vi "Write.vi"(8 "error in (no error)":errorcluster, 10 "write buffer":string, 11 "MODBUS in":refnum<class "PL Modbus Client.lvclass">) -> (0 "error out":errorcluster, 3 "MODBUS out":refnum<class "PL Modbus Client.lvclass">)   [LabVIEW 2015, in "PL Modbus Client.lvclass"]
doc: "Writes bytes to specified interface."
uses:
  PL Modbus Client.lvclass
  PL Modbus Client.lvclass/PL Modbus Client.ctl
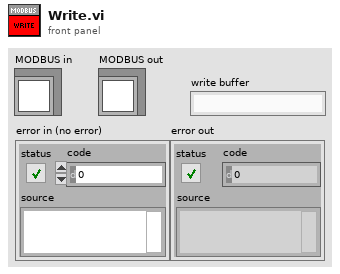
[diagram p1: front panel]
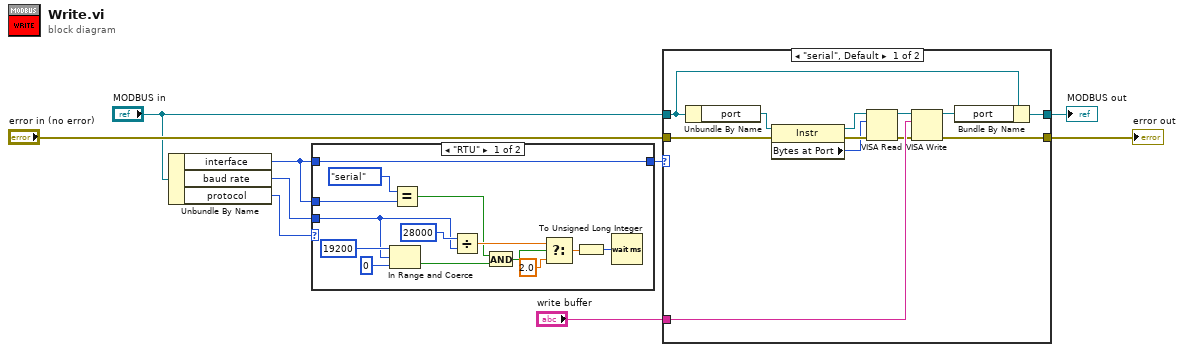
[diagram p0: block diagram]
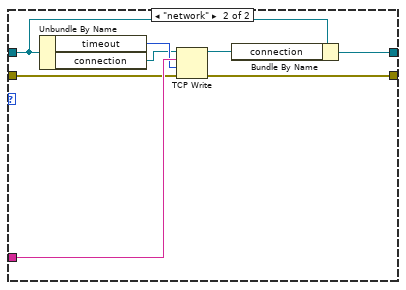
[diagram p3: hidden frame]
diagram:
  n1 = Unbundle By Name("MODBUS in") -> ("interface"=w4:enum16{"serial", "network"}, "baud rate"=w5:u32, "protocol"=w6:enum16{"RTU", "ASCII", "TCP"})
  n2 = case shown="\"RTU\"" w6 {
    tunnel: w5 -> [w13 _]
    tunnel: w4 -> [w12 _]
    tunnel: w4 -> [w10 w24]
    tunnel: [w10 w24] -> w3
    frame "RTU" {
      n3 = In Range and Coerce(upper limit=u32 19200, x=w13, lower limit=u32 0) -> (In Range?=w15:bool)  [unwired: 1 out]
      n4 = Equal?(x=enum16{"serial", "TCP"}."serial", y=w12) -> (x = y?=w16:bool)
      n5 = Divide(x=u32 28000, y=w13) -> (x/y=w19:dbl)
      n6 = And(x=w16, y=w15) -> (x .and. y?=w14:bool)
      n7 = Select(t=w19, s=w14, f=2.0) -> (s? t:f=w18:dbl)
      n8 = To Unsigned Long Integer(number=w18) -> (unsigned 32bit integer=w11:u32)
      n9 = Wait (ms)(milliseconds to wait=w11) -> ()  [unwired: 1 out]
    }
    frame "ASCII", Default {
    }
  }
  n10 = case shown="\"serial\", Default" w3 {
    tunnel: "MODBUS in" -> [w36 w40]
    tunnel: "error in (no error)" -> [w26 w38]
    tunnel: [w34 w44] -> w9
    tunnel: [w33 w43] -> w8
    tunnel: "write buffer" -> [w32 w41]
    frame "serial", Default {
      n11 = Unbundle By Name(w36) -> ("port"=w31:refnum<visa-resource-name>)
      n12 = property class="Instr"(reference=w31, error in=w26) -> (reference out=w29:refnum<visa-resource-name>, error out=w28:errorcluster, "Bytes at Port"=w27:u32)
      n13 = VISA Read(VISA resource name=w29, byte count=w27, error in (no error)=w28) -> (VISA resource name out=w30:refnum<visa-resource-name>, error out=w25:errorcluster)  [unwired: 2 out]
      n14 = VISA Write(VISA resource name=w30, write buffer=w32, error in (no error)=w25) -> (VISA resource name out=w35:refnum<visa-resource-name>, error out=w33:errorcluster)  [unwired: 1 out]
      n15 = Bundle By Name(cluster=w36, "port"=w35) -> (w34:refnum<class "PL Modbus Client.lvclass">)
    }
    frame "network" {
      n16 = Unbundle By Name(w40) -> ("timeout"=w39:u32, "connection"=w37:refnum<k5>)
      n17 = TCP Write(connection ID=w37, data in=w41, error in (no error)=w38, 9:w39) -> (connection ID out=w42:refnum<k5>, error out=w43:errorcluster)  [unwired: 1 out]
      n18 = Bundle By Name(cluster=w40, "connection"=w42) -> (w44:refnum<class "PL Modbus Client.lvclass">)
    }
  }
  "MODBUS out" <- w9
  "error out" <- w8
